vi "Write configuration.vi"(8 "error in (no error)":errorcluster, 10 "configuration":refnum<class "CEF_serializable configuration.lvclass">, 11 "HiPOT Instrument":refnum<class "HiPOT Instrument.lvclass">) -> (0 "error out":errorcluster, 3 "HiPOT Instrument out":refnum<class "HiPOT Instrument.lvclass">)   [LabVIEW 2025, in "HiPOT.lvlib" / "HiPOT Instrument.lvclass"]
uses:
  HiPOT Instrument.lvclass
  Users/Public/Documents/Sandia National Labs/TSS Plugin/CEF.lvlibp/serializable configuration/CEF_serializable configuration.lvclass
  HiPOT configuration/HiPOT configuration.lvclass
  HiPOT Instrument.lvclass/HiPOT Instrument.ctl
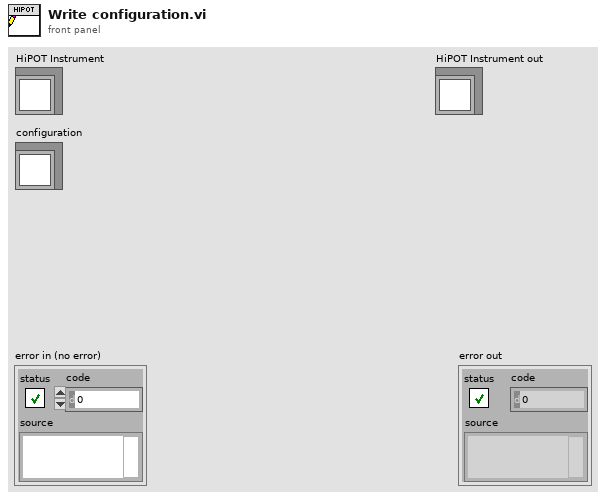
[diagram p1: front panel]
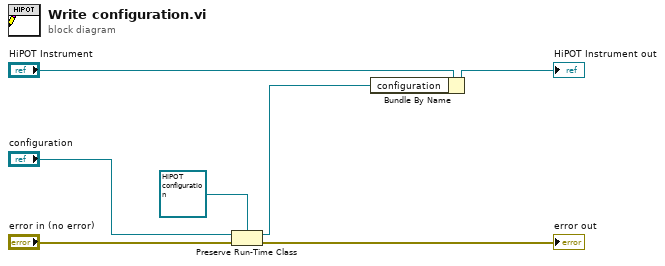
[diagram p0: block diagram]
diagram:
  n1 = Preserve Run-Time Class(object in="configuration", error in="error in (no error)", 2:refnum<class "HiPOT configuration.lvclass"> refnum ("Digitizer.lvlib:Digitizer configuration.lvclass")) -> (object out=w4:refnum<class "HiPOT configuration.lvclass">, error out=→"error out":errorcluster)
  n2 = Bundle By Name(cluster="HiPOT Instrument", "configuration"=w4) -> (→"HiPOT Instrument out":refnum<class "HiPOT Instrument.lvclass">)
